vi "Auto State Machine.vi"   [LabVIEW 2013]
uses:
  typedefs/State Machine/singleUseSubstate.ctl
  typedefs/fg_typedef.ctl
  typedefs/State Machine/subStates.ctl
  typedefs/DevRef Type.ctl
panel:
  # "A State Machine to Handle One or Two Ball Autonomous"
types:
  T1 = typedef "fg_typedef.ctl" = enum16{"Get", "Set"}
  T2 = typedef "singleUseSubstate.ctl" = enum16{"null", "wait", "shift high", "shift low", "extend shooter", "retract shooter", "latch", "unlatch", "end"}
  T3 = typedef "DevRef Type.ctl" = enum16{"Shooter Solenoid", "Latch Solenoid", "Right Up Sensor", "Right Down Sensor", "Hold Sensor", "2 Ball Switch", "Arm Encoder"}
  T4 = typedef "subStates.ctl" = enum16{"null", "wait", "driver control", "auto", "manual override", "hold position", "rotate", "pickup", "pass", "load", "goto shoot", "shoot high goal", "shoot low goal", "cancel arm", "cancel shooter", "end", "test"}
  T5 = typedef "WPI_DigitalInputDevRef.ctl" = cluster{"DevStatus":errorcluster, "DIO Channel":T6, "Digital Module":T7}
  T6 = typedef "FPGA_DIOChannel.ctl" = enum8{"DIO 1", "DIO 2", "DIO 3", "DIO 4", "DIO 5", "DIO 6", "DIO 7", "DIO 8", "DIO 9", "DIO 10", "DIO 11", "DIO 12", "DIO 13", "DIO 14", "Invalid"}
  T7 = typedef "FPGA_TypedefDigitalModule.ctl" = enum16{"Digital Module 1", "Digital Module 2"}
  T8 = typedef "vision data.ctl" = cluster{"x":dbl, "y":dbl, "area":dbl, "width":dbl, "height":dbl, "Hot Goal Present?":bool, "distance":dbl}
  T9 = typedef "WPI_EncoderDevRef.ctl" = cluster{"DevStatus":errorcluster, "EncoderIndex":T10, "CounterIndex":T11, "DistancePerCount":dbl, "Decoding Type":T12}
  T10 = typedef "FPGA_EncoderIdx.ctl" = enum8{"Enc 0", "Enc 1", "Enc 2", "Enc 3", "Invalid"}
  T11 = typedef "FPGA_CounterCtrSystemIndex.ctl" = enum8{"Ctr 0", "Ctr 1", "Ctr 2", "Ctr 3", "Ctr 4", "Ctr 5", "Ctr 6", "Ctr 7", "Invalid"}
  T12 = typedef "WPI_EncoderType.ctl" = enum16{"1x", "2x", "4x"}
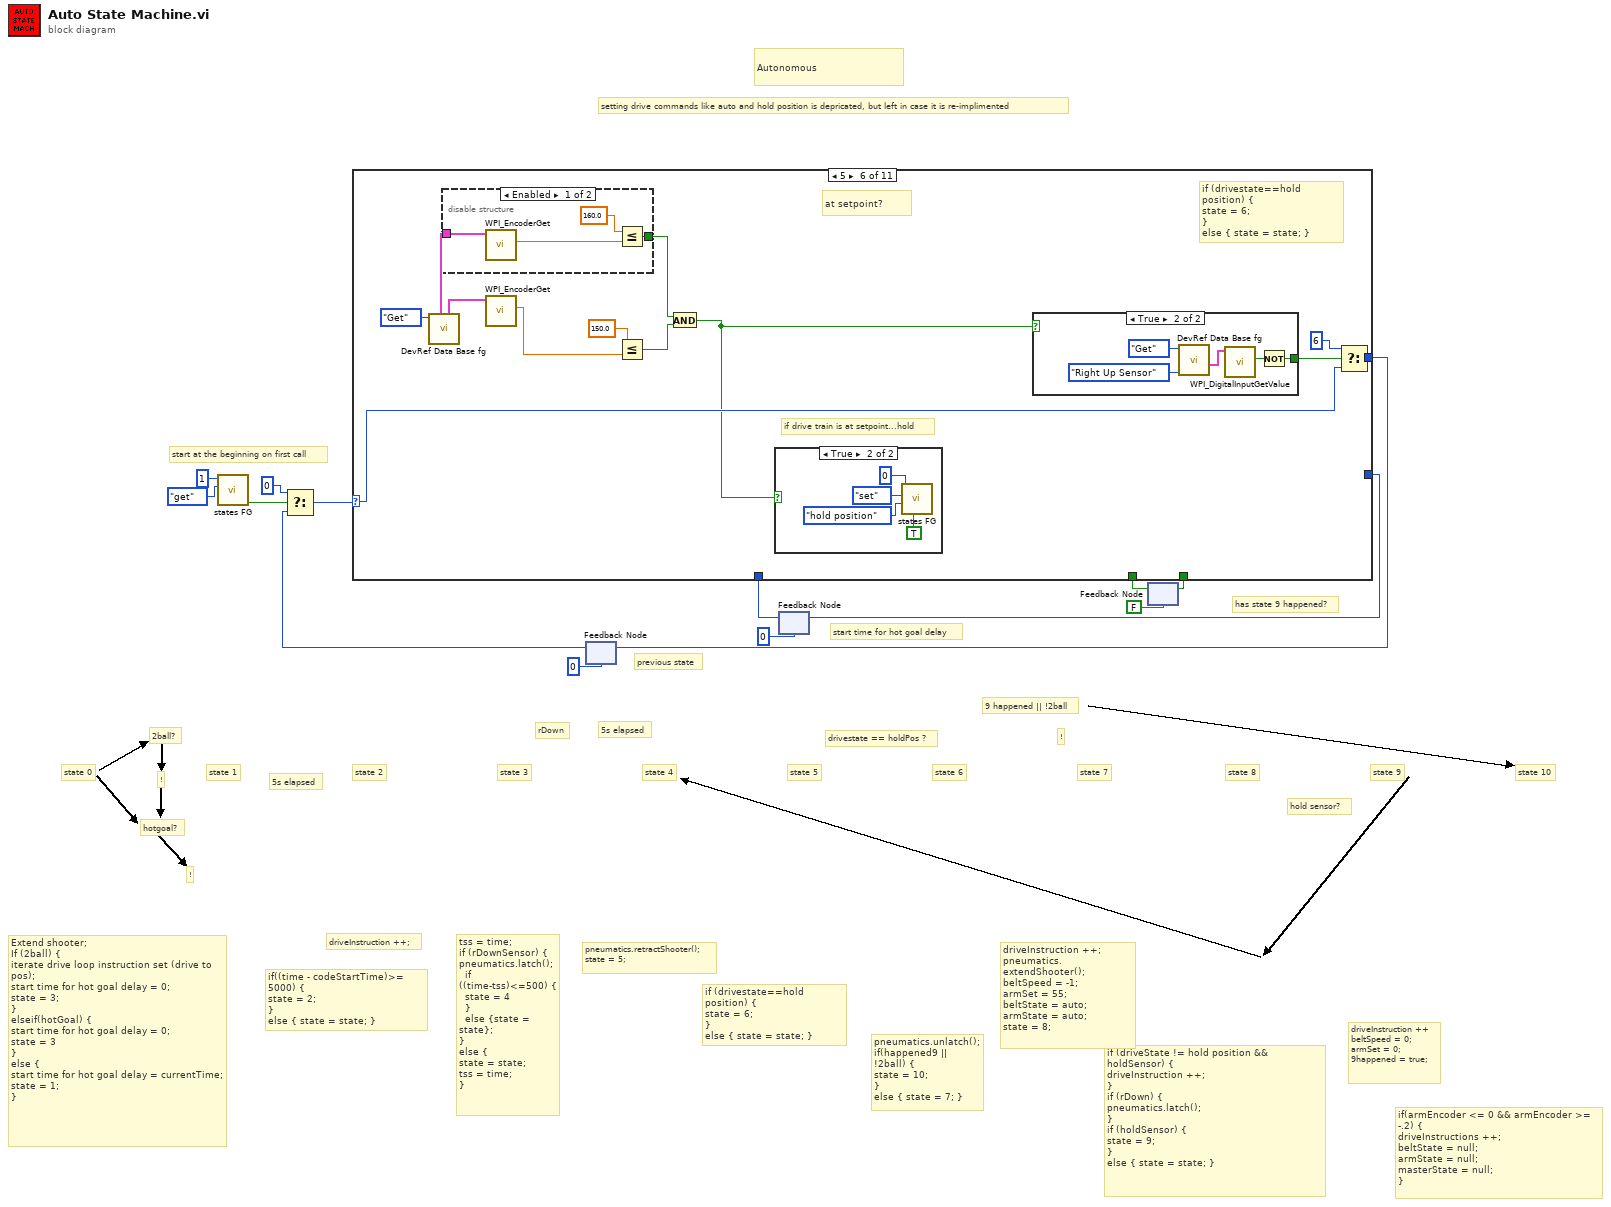
[diagram p0: block diagram]
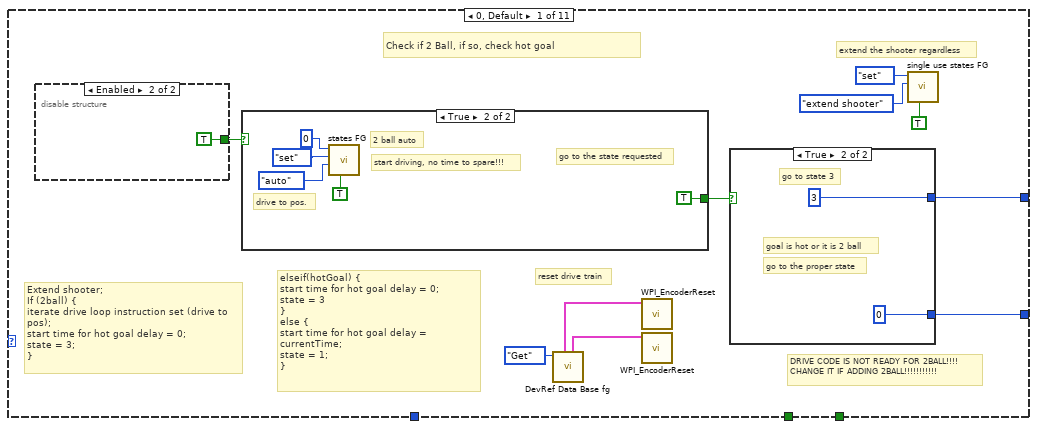
[diagram p2: hidden frame]
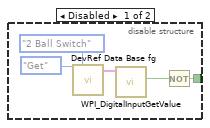
[diagram p3: hidden frame]
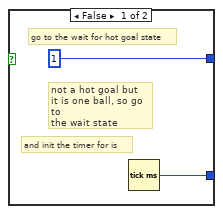
[diagram p4: hidden frame]
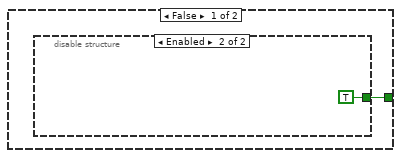
[diagram p5: hidden frame]
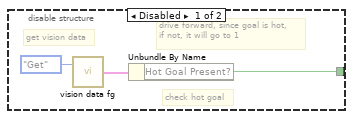
[diagram p6: hidden frame]
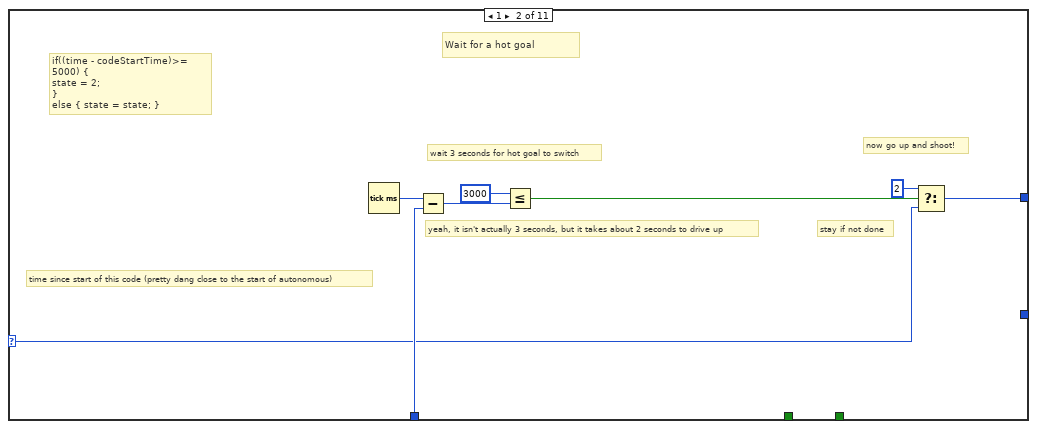
[diagram p7: hidden frame]
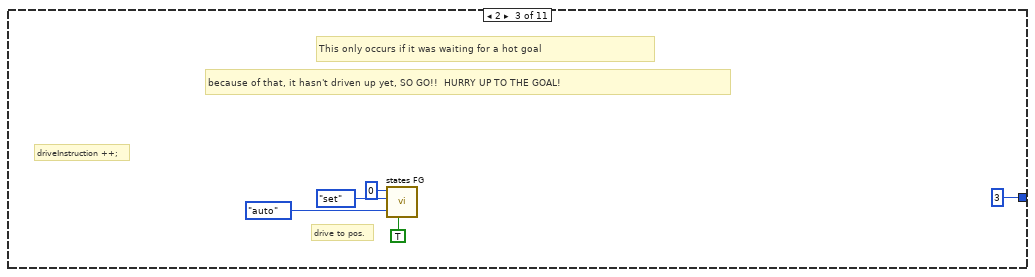
[diagram p8: hidden frame]
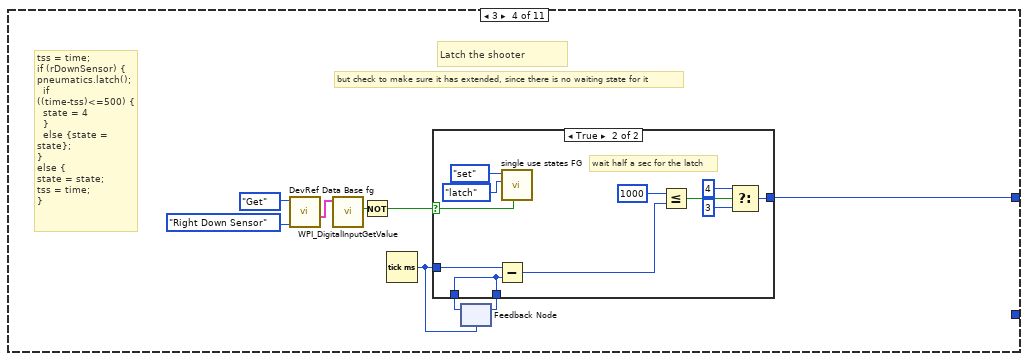
[diagram p9: hidden frame]
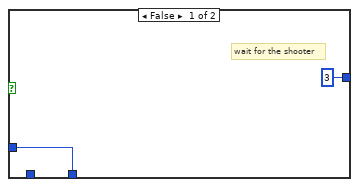
[diagram p10: hidden frame]
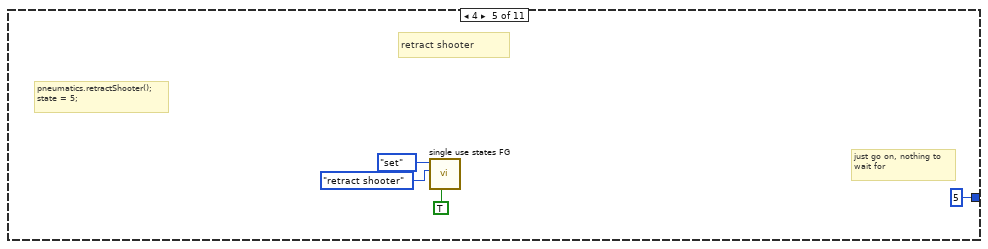
[diagram p11: hidden frame]
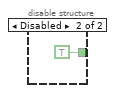
[diagram p12: hidden frame]
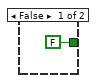
[diagram p13: hidden frame]
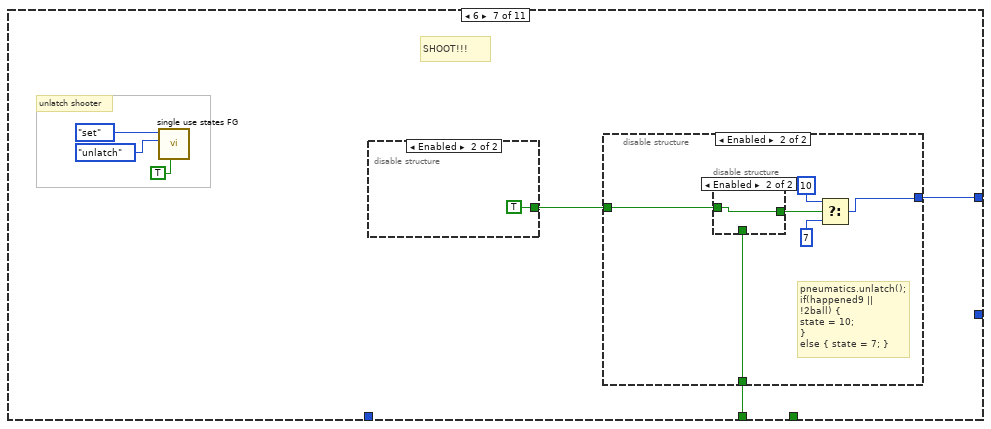
[diagram p15: hidden frame]
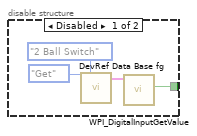
[diagram p16: hidden frame]
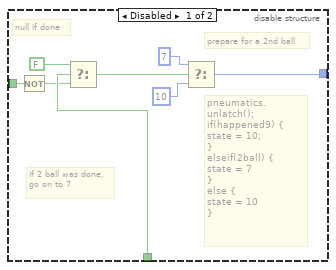
[diagram p17: hidden frame]
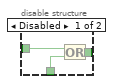
[diagram p18: hidden frame]
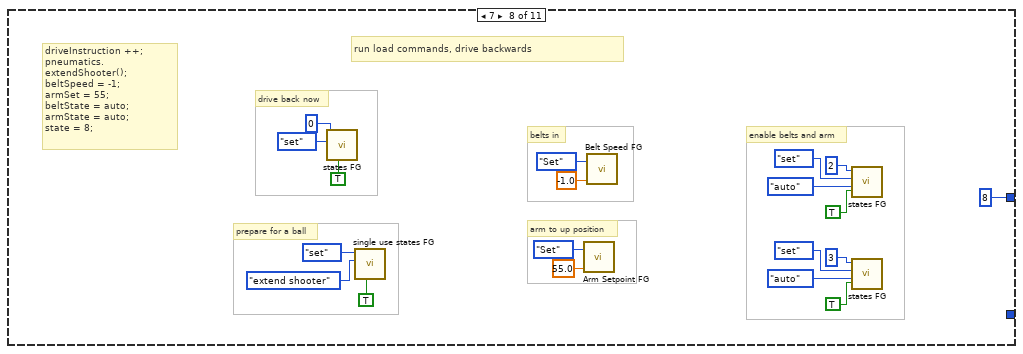
[diagram p19: hidden frame]
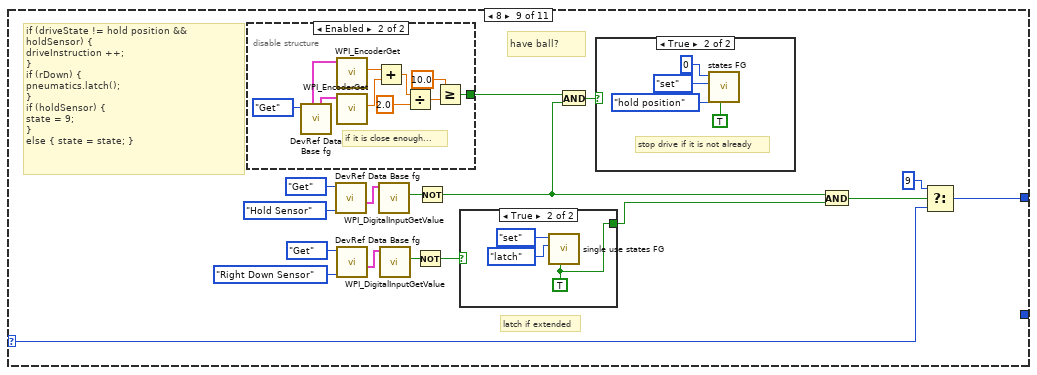
[diagram p20: hidden frame]
diagram:
  # "setting drive commands like auto and hold position is depricated, but left in case it is re-implimented"
  # "if(armEncoder <= 0 && armEncoder >= -.2) {\ndriveInstructions ++;\nbeltState = null;\narmState = null;\nmasterState = null;\n}"
  # "driveInstruction ++\nbeltSpeed = 0;\narmSet = 0;\n9happened = true;"
  # "if (driveState != hold position && holdSensor) {\ndriveInstruction ++;\n}\nif (rDown) {\npneumatics.latch();\n}\nif (holdSensor) {\nstate = 9;\n}\nelse { state = state; }"
  # "driveInstruction ++;\npneumatics.extendShooter();\nbeltSpeed = -1;\narmSet = 55;\nbeltState = auto;\narmState = auto;\nstate = 8;"
  # "pneumatics.unlatch();\nif(happened9 || !2ball) {\nstate = 10;\n}\nelse { state = 7; }"
  # "if (drivestate==hold position) {\nstate = 6;\n}\nelse { state = state; }"
  # "pneumatics.retractShooter();\nstate = 5;"
  # "tss = time;\nif (rDownSensor) {\npneumatics.latch();\n  if ((time-tss)<=500) {\n  state = 4\n  }\n  else {state = state};\n}\nelse {\nstate = state;\ntss = time;\n}"
  # "driveInstruction ++;"
  # "if((time - codeStartTime)>= 5000) {\nstate = 2;\n}\nelse { state = state; }"
  # "Extend shooter;\nIf (2ball) {\niterate drive loop instruction set (drive to pos);\nstart time for hot goal delay = 0;\nstate = 3;\n}\nelseif(hotGoal) {\nstart time for hot goal delay = 0;\nstate = 3\n}\nelse {\nstart time for hot goal delay = currentTime;\nstate = 1;\n}"
  # "hold sensor?"
  # "!"
  # "9 happened || !2ball"
  # "drivestate == holdPos ?"
  # "5s elapsed"
  # "rDown"
  # "5s elapsed"
  # "!"
  # "hotgoal?"
  # "!"
  # "state 10"
  # "2ball?"
  # "state 9"
  # "state 8"
  # "state 7"
  # "state 6"
  # "state 5"
  # "state 4"
  # "state 3"
  # "state 2"
  # "state 1"
  # "state 0"
  # "has state 9 happened?"
  # "start time for hot goal delay"
  # "previous state"
  # "start at the beginning on first call"
  # "Autonomous"
  n1 = call "states FG.vi"("menu (get)"=enum16{"set", "get"}."get", "Loop ID"=1) -> ("first call?"=w9:bool)  [unwired: 6 in, 3 out]
  n2 = feedback #1(u8 0) -> (w10:u8)
  n3 = Select(t=u8 0, s=w9, f=w10) -> (s? t:f=w12:u8)
  n4 = feedback #2(u32 0 ("millisecond timer value")) -> (w4:u32)
  n5 = feedback #3(FALSE) -> (w2:bool)
  n6 = case shown="5" w12 {
    selector: w12 -> [_ w45 _ _ _ w95 _ _ w174 _ w210]
    tunnel: [w23 w46 u8 3 ("t") w60 u8 5 ("t") w93 w116 u8 8 ("t") w173 u8 4 ("t") w210] -> w7
    tunnel: [w22 _ _ _ _ _ _ _ _ _ _] -> w6
    tunnel: w4 -> [_ w49 _ _ _ _ _ _ _ _ _]
    tunnel: [_ _ _ _ _ _ _ _ _ TRUE _] -> w3
    tunnel: w2 -> [_ _ _ _ _ _ w112 _ _ _ _]
    frame 0, Default {
      # "DRIVE CODE IS NOT READY FOR 2BALL!!!!\nCHANGE IT IF ADDING 2BALL!!!!!!!!!!!"
      # "reset drive train"
      # "extend the shooter regardless"
      # "elseif(hotGoal) {\nstart time for hot goal delay = 0;\nstate = 3\n}\nelse {\nstart time for hot goal delay = currentTime;\nstate = 1;\n}"
      # "Extend shooter;\nIf (2ball) {\niterate drive loop instruction set (drive to pos);\nstart time for hot goal delay = 0;\nstate = 3;\n}"
      # "Check if 2 Ball, if so, check hot goal"
      n7 = disable-structure shown="Enabled" {
        disable-tunnel: [w25 TRUE] -> w21
        frame Disabled {
          n8 = call "DevRef Data Base fg.vi"(0:fg_typedef."Get" ("Menu"), 10:DevRef_Type."2 Ball Switch" ("DevRef to Get")) -> ("Selected Sensor"=w27:T5)  [unwired: 22 in, 3 out]
          n9 = call <vilib>:"WPI_DigitalInputGetValue.vi"("DigitalInputDevRef"=w27) -> ("Value"=w26:bool)  [unwired: 8 in, 2 out]
          n10 = Not(x=w26) -> (.not. x?=w25:bool)
        }
        frame Enabled {
        }
      }
      n11 = case shown="True" w21 {
        tunnel: [w35 TRUE ("Hot Goal Present?")] -> w24
        frame False {
          n12 = disable-structure shown="Enabled" {
            disable-tunnel: [w36 TRUE ("Hot Goal Present?")] -> w35
            frame Disabled {
              # "drive forward, since goal is hot,\nif not, it will go to 1"
              # "check hot goal"
              # "get vision data"
              n13 = call "vision data fg.vi"("Menu"=fg_typedef."Get") -> ("Output"=w37:T8)  [unwired: 1 in]
              n14 = Unbundle By Name(w37) -> ("Hot Goal Present?"=w36:bool)
            }
            frame Enabled {
            }
          }
        }
        frame True {
          # "go to the state requested"
          # "drive to pos."
          # "start driving, no time to spare!!!"
          # "2 ball auto"
          n15 = call "states FG.vi"("exit in"=TRUE, "subState in"=subStates."auto", "menu (get)"=enum16{"set", "get"}."set", "Loop ID"=0) -> ()  [unwired: 4 in, 4 out]
        }
      }
      n16 = call "DevRef Data Base fg.vi"("Menu"=fg_typedef."Get") -> ("right drive encoder"=w15:T9, "left drive encoder"=w16:T9)  [unwired: 3 in, 4 out]
      n17 = call <vilib>:"WPI_EncoderReset.vi"("EncoderDevRef"=w16) -> ()  [unwired: 9 in, 2 out]
      n18 = call <vilib>:"WPI_EncoderReset.vi"("EncoderDevRef"=w15) -> ()  [unwired: 9 in, 2 out]
      n19 = case shown="True" w24 {
        tunnel: [u8 1 ("f") u8 3] -> w23
        tunnel: [w32 u32 0 ("millisecond timer value")] -> w22
        frame False {
          # "go to the wait for hot goal state"
          # "and init the timer for is"
          # "not a hot goal but\nit is one ball, so go to\nthe wait state"
          n20 = Tick Count (ms)() -> (millisecond timer value=w32:u32)
        }
        frame True {
          # "go to state 3"
          # "go to the proper state"
          # "goal is hot or it is 2 ball"
        }
      }
      n21 = call "single use states FG.vi"("exit in"=TRUE, "substate"=singleUseSubstate."extend shooter", "menu (get)"=enum16{"set", "get"}."set") -> ()  [unwired: 5 in, 4 out]
    }
    frame 1 {
      # "yeah, it isn't actually 3 seconds, but it takes about 2 seconds to drive up"
      # "if((time - codeStartTime)>= 5000) {\nstate = 2;\n}\nelse { state = state; }"
      # "now go up and shoot!"
      # "stay if not done"
      # "time since start of this code (pretty dang close to the start of autonomous)"
      # "wait 3 seconds for hot goal to switch"
      # "Wait for a hot goal"
      n22 = Tick Count (ms)() -> (millisecond timer value=w50:u32)
      n23 = Subtract(x=w50, y=w49) -> (x-y=w52:u32)
      n24 = Less Or Equal?(x=u32 3000, y=w52) -> (x <= y?=w48:bool)
      n25 = Select(t=u8 2, s=w48, f=w45) -> (s? t:f=w46:u8)
    }
    frame 2 {
      # "driveInstruction ++;"
      # "drive to pos."
      # "because of that, it hasn't driven up yet, SO GO!!  HURRY UP TO THE GOAL!"
      # "This only occurs if it was waiting for a hot goal"
      n26 = call "states FG.vi"("exit in"=TRUE, "subState in"=subStates."auto", "menu (get)"=enum16{"set", "get"}."set", "Loop ID"=0) -> ()  [unwired: 4 in, 4 out]
    }
    frame 3 {
      # "tss = time;\nif (rDownSensor) {\npneumatics.latch();\n  if ((time-tss)<=500) {\n  state = 4\n  }\n  else {state = state};\n}\nelse {\nstate = state;\ntss = time;\n}"
      # "but check to make sure it has extended, since there is no waiting state for it"
      # "Latch the shooter"
      n27 = call "DevRef Data Base fg.vi"("DevRef to Get"=DevRef_Type."Right Down Sensor", "Menu"=fg_typedef."Get") -> ("Selected Sensor"=w66:T5)  [unwired: 2 in, 5 out]
      n28 = call <vilib>:"WPI_DigitalInputGetValue.vi"("DigitalInputDevRef"=w66) -> ("Value"=w65:bool)  [unwired: 8 in, 2 out]
      n29 = Not(x=w65) -> (.not. x?=w64:bool)
      n30 = Tick Count (ms)() -> (millisecond timer value=w61:u32)
      n31 = feedback #4(w61) -> (w62:u32)
      n32 = case shown="True" w64 {
        selector: w64 -> [_ w75]
        tunnel: [w67 w77] -> w63
        tunnel: w62 -> [_ w77]
        tunnel: w61 -> [w67 w76]
        tunnel: [u8 3 ("f") w70] -> w60
        frame False {
          # "wait for the shooter"
        }
        frame True {
          # "wait half a sec for the latch"
          n33 = Subtract(x=w76, y=w77) -> (x-y=w72:u32)
          n34 = call "single use states FG.vi"("exit in"=w75, "substate"=singleUseSubstate."latch", "menu (get)"=enum16{"set", "get"}."set") -> ()  [unwired: 5 in, 4 out]
          n35 = Less Or Equal?(x=u32 1000, y=w72) -> (x <= y?=w69:bool)
          n36 = Select(t=u8 4, s=w69, f=u8 3) -> (s? t:f=w70:u8)
        }
      }
      n37 = feedback-in #4(w63) -> ()
    }
    frame 4 {
      # "pneumatics.retractShooter();\nstate = 5;"
      # "just go on, nothing to\nwait for"
      # "retract shooter"
      n38 = call "single use states FG.vi"("exit in"=TRUE, "substate"=singleUseSubstate."retract shooter", "menu (get)"=enum16{"set", "get"}."set") -> ()  [unwired: 5 in, 4 out]
    }
    frame 5 {
      # "if drive train is at setpoint...hold"
      # "if (drivestate==hold position) {\nstate = 6;\n}\nelse { state = state; }"
      # "at setpoint?"
      n39 = call "DevRef Data Base fg.vi"("Menu"=fg_typedef."Get") -> ("right drive encoder"=w90:T9, "left drive encoder"=w89:T9)  [unwired: 3 in, 4 out]
      n40 = disable-structure shown="Enabled" {
        disable-tunnel: w89 -> [w98 _]
        disable-tunnel: [w96 TRUE] -> w86
        frame Enabled {
          n41 = call <vilib>:"WPI_EncoderGet.vi"("EncoderDevRef"=w98) -> ("Distance"=w97:dbl)  [unwired: 5 in, 5 out]
          n42 = Less Or Equal?(x=160.0, y=w97) -> (x <= y?=w96:bool)
        }
        frame Disabled {
        }
      }
      n43 = call <vilib>:"WPI_EncoderGet.vi"("EncoderDevRef"=w90) -> ("Distance"=w87:dbl)  [unwired: 5 in, 5 out]
      n44 = Less Or Equal?(x=150.0, y=w87) -> (x <= y?=w85:bool)
      n45 = And(x=w86, y=w85) -> (x .and. y?=w84:bool)
      n46 = case shown="True" w84 {
        frame False {
        }
        frame True {
          n47 = call "states FG.vi"("exit in"=TRUE, "subState in"=subStates."hold position" ("y"), "menu (get)"=enum16{"set", "get"}."set", "Loop ID"=0) -> ()  [unwired: 4 in, 4 out]
        }
      }
      n48 = case shown="True" w84 {
        tunnel: [FALSE w104] -> w92
        frame False {
        }
        frame True {
          n49 = call "DevRef Data Base fg.vi"("DevRef to Get"=DevRef_Type."Right Up Sensor", "Menu"=fg_typedef."Get") -> ("Selected Sensor"=w106:T5)  [unwired: 2 in, 5 out]
          n50 = call <vilib>:"WPI_DigitalInputGetValue.vi"("DigitalInputDevRef"=w106) -> ("Value"=w105:bool)  [unwired: 8 in, 2 out]
          n51 = Not(x=w105) -> (.not. x?=w104:bool)
        }
      }
      n52 = Select(t=u8 6, s=w92, f=w95) -> (s? t:f=w93:u8)
    }
    frame 6 {
      # "unlatch shooter"
      # "SHOOT!!!"
      n53 = call "single use states FG.vi"("exit in"=TRUE, "substate"=singleUseSubstate."unlatch", "menu (get)"=enum16{"set", "get"}."set") -> ()  [unwired: 5 in, 4 out]
      n54 = disable-structure shown="Enabled" {
        disable-tunnel: [w117 TRUE ("Value")] -> w111
        frame Disabled {
          n55 = call "DevRef Data Base fg.vi"(0:fg_typedef."Get" ("Menu"), 10:DevRef_Type."2 Ball Switch" ("DevRef to Get")) -> ("Selected Sensor"=w118:T5)  [unwired: 22 in, 3 out]
          n56 = call <vilib>:"WPI_DigitalInputGetValue.vi"("DigitalInputDevRef"=w118) -> ("Value"=w117:bool)  [unwired: 8 in, 2 out]
        }
        frame Enabled {
        }
      }
      n57 = disable-structure shown="Enabled" {
        disable-tunnel: [w128 w131] -> w116
        disable-tunnel: w112 -> [w126 w135]
        disable-tunnel: w111 -> [w125 w130]
        frame Disabled {
          # "pneumatics.unlatch();\nif(happened9) {\nstate = 10;\n}\nelseif(2ball) {\nstate = 7\n}\nelse {\nstate = 10\n}"
          # "if 2 ball was done,\ngo on to 7"
          # "prepare for a 2nd ball"
          # "null if done"
          n58 = Not(x=w125) -> (.not. x?=w122:bool)
          n59 = Select(t=FALSE, s=w126, f=w122) -> (s? t:f=w123:bool)
          n60 = Select(t=u8 7, s=w123, f=u8 10 ("t")) -> (s? t:f=w128:u8)
        }
        frame Enabled {
          # "pneumatics.unlatch();\nif(happened9 || !2ball) {\nstate = 10;\n}\nelse { state = 7; }"
          n61 = disable-structure shown="Enabled" {
            disable-tunnel: w135 -> [w138 _]
            disable-tunnel: [w137 w139] -> w134
            disable-tunnel: w130 -> [w136 w139]
            frame Disabled {
              n62 = Or(x=w136, y=w138) -> (x .or. y?=w137:bool)
            }
            frame Enabled {
            }
          }
          n63 = Select(t=u8 10, s=w134, f=u8 7 ("t")) -> (s? t:f=w131:u8)
        }
      }
    }
    frame 7 {
      # "drive back now"
      # "prepare for a ball"
      # "arm to up position"
      # "enable belts and arm"
      # "driveInstruction ++;\npneumatics.extendShooter();\nbeltSpeed = -1;\narmSet = 55;\nbeltState = auto;\narmState = auto;\nstate = 8;"
      # "belts in"
      # "run load commands, drive backwards"
      n64 = call "states FG.vi"("exit in"=TRUE, "menu (get)"=enum16{"set", "get"}."set", "Loop ID"=0) -> ()  [unwired: 5 in, 4 out]
      n65 = call "single use states FG.vi"("exit in"=TRUE, "substate"=singleUseSubstate."extend shooter", "menu (get)"=enum16{"set", "get"}."set") -> ()  [unwired: 5 in, 4 out]
      n66 = call "Arm Setpoint FG.vi"("Setpoint In"=55.0, "Menu"=fg_typedef."Set") -> ()  [unwired: 1 out]
      n67 = call "Belt Speed FG.vi"("Speed In"=-1.0, "Menu"=fg_typedef."Set") -> ()  [unwired: 1 out]
      n68 = call "states FG.vi"("exit in"=TRUE, "subState in"=subStates."auto", "menu (get)"=enum16{"set", "get"}."set", "Loop ID"=2) -> ()  [unwired: 4 in, 4 out]
      n69 = call "states FG.vi"("exit in"=TRUE, "subState in"=subStates."auto", "menu (get)"=enum16{"set", "get"}."set", "Loop ID"=3) -> ()  [unwired: 4 in, 4 out]
    }
    frame 8 {
      # "if (driveState != hold position && holdSensor) {\ndriveInstruction ++;\n}\nif (rDown) {\npneumatics.latch();\n}\nif (holdSensor) {\nstate = 9;\n}\nelse { state = state; }"
      # "latch if extended"
      # "have ball?"
      n70 = disable-structure shown="Enabled" {
        disable-tunnel: [w176 w181] -> w168
        frame Disabled {
          n71 = call "states FG.vi"("menu (get)"=enum16{"set", "get"}."get", "Loop ID"=0) -> ("subState out"=w178:T4)  [unwired: 6 in, 3 out]
          n72 = Not Equal?(x=w178, y=subStates."hold position") -> (x != y?=w176:bool)
        }
        frame Enabled {
          # "if it is close enough..."
          n73 = call "DevRef Data Base fg.vi"("Menu"=fg_typedef."Get") -> ("right drive encoder"=w183:T9, "left drive encoder"=w182:T9)  [unwired: 3 in, 4 out]
          n74 = call <vilib>:"WPI_EncoderGet.vi"("EncoderDevRef"=w182) -> ("Distance"=w190:dbl)  [unwired: 5 in, 5 out]
          n75 = call <vilib>:"WPI_EncoderGet.vi"("EncoderDevRef"=w183) -> ("Distance"=w189:dbl)  [unwired: 5 in, 5 out]
          n76 = Add(x=w190, y=w189) -> (x+y=w188:dbl)
          n77 = Divide(x=w188, y=2.0) -> (x/y=w186:dbl)
          n78 = Greater Or Equal?(x=10.0, y=w186) -> (x >= y?=w181:bool)
        }
      }
      n79 = call "DevRef Data Base fg.vi"("DevRef to Get"=DevRef_Type."Hold Sensor", "Menu"=fg_typedef."Get") -> ("Selected Sensor"=w172:T5)  [unwired: 2 in, 5 out]
      n80 = call "DevRef Data Base fg.vi"("DevRef to Get"=DevRef_Type."Right Down Sensor", "Menu"=fg_typedef."Get") -> ("Selected Sensor"=w167:T5)  [unwired: 2 in, 5 out]
      n81 = call <vilib>:"WPI_DigitalInputGetValue.vi"("DigitalInputDevRef"=w172) -> ("Value"=w171:bool)  [unwired: 8 in, 2 out]
      n82 = call <vilib>:"WPI_DigitalInputGetValue.vi"("DigitalInputDevRef"=w167) -> ("Value"=w166:bool)  [unwired: 8 in, 2 out]
      n83 = Not(x=w166) -> (.not. x?=w165:bool)
      n84 = Not(x=w171) -> (.not. x?=w169:bool)
      n85 = case shown="True" w165 {
        tunnel: [FALSE w192] -> w163
        frame False {
          # "wait.."
        }
        frame True {
          w192 = TRUE
          n86 = call "single use states FG.vi"("exit in"=w192, "substate"=singleUseSubstate."latch", "menu (get)"=enum16{"set", "get"}."set") -> ()  [unwired: 5 in, 4 out]
        }
      }
      n87 = And(x=w168, y=w169) -> (x .and. y?=w170:bool)
      n88 = case shown="True" w170 {
        frame False {
        }
        frame True {
          # "stop drive if it is not already"
          n89 = call "states FG.vi"("exit in"=TRUE, "subState in"=subStates."hold position", "menu (get)"=enum16{"set", "get"}."set", "Loop ID"=0) -> ()  [unwired: 4 in, 4 out]
        }
      }
      n90 = And(x=w169, y=w163) -> (x .and. y?=w164:bool)
      n91 = Select(t=u8 9, s=w164, f=w174) -> (s? t:f=w173:u8)
    }
    frame 9 {
      # "driveInstruction ++\nbeltSpeed = 0;\narmSet = 0;\n9happened = true;"
      # "arm down"
      # "belts off"
      # "sends drive into auto state (due to autonomous code setup)"
      # "drive to pos."
      # "drive forward, arm down, belts off"
      n92 = call "states FG.vi"("exit in"=TRUE, "subState in"=subStates."auto", "menu (get)"=enum16{"set", "get"}."set", "Loop ID"=0) -> ()  [unwired: 4 in, 4 out]
      n93 = call "Arm Setpoint FG.vi"("Setpoint In"=0.0, "Menu"=fg_typedef."Set") -> ()  [unwired: 1 out]
      n94 = call "Belt Speed FG.vi"("Speed In"=0.0, "Menu"=fg_typedef."Set") -> ()  [unwired: 1 out]
    }
    frame 10 {
      # "if(armEncoder <= 0 && armEncoder >= -.2) {\ndriveInstructions ++;\nbeltState = null;\narmState = null;\nmasterState = null;\n}"
      # "null all the things"
      n95 = disable-structure shown="Enabled" {
        disable-tunnel: [w211 TRUE] -> w209
        frame Disabled {
          n96 = call "DevRef Data Base fg.vi"(0:fg_typedef."Get" ("Menu"), 10:DevRef_Type."Arm Encoder" ("DevRef to Get")) -> ("Selected Encoder"=w215:T9)  [unwired: 22 in, 3 out]
          n97 = call <vilib>:"WPI_EncoderGet.vi"("EncoderDevRef"=w215) -> ("Distance"=w214:dbl)  [unwired: 5 in, 5 out]
          n98 = In Range and Coerce(upper limit=1.0, x=w214, lower limit=-0.4) -> (In Range?=w211:bool)  [unwired: 1 out]
        }
        frame Enabled {
        }
      }
      n99 = case shown="True" w209 {
        frame False {
        }
        frame True {
          # "null things"
          n100 = call "states FG.vi"("exit in"=TRUE, "subState in"=subStates."null", "menu (get)"=enum16{"set", "get"}."set", "Loop ID"=0) -> ()  [unwired: 4 in, 4 out]
          n101 = call "states FG.vi"("exit in"=TRUE, "subState in"=subStates."null", "menu (get)"=enum16{"set", "get"}."set", "Loop ID"=1) -> ()  [unwired: 4 in, 4 out]
          n102 = call "states FG.vi"("exit in"=TRUE, "subState in"=subStates."null", "menu (get)"=enum16{"set", "get"}."set", "Loop ID"=2) -> ()  [unwired: 4 in, 4 out]
          n103 = call "states FG.vi"("exit in"=TRUE, "subState in"=subStates."null", "menu (get)"=enum16{"set", "get"}."set", "Loop ID"=3) -> ()  [unwired: 4 in, 4 out]
        }
      }
    }
  }
  n104 = feedback-in #1(w7) -> ()
  n105 = feedback-in #2(w6) -> ()
  n106 = feedback-in #3(w3) -> ()
